vi "Check Knobs.vi"(5 "Knobs Present":bool[](array[boolean]), 7 "Number of Knobs":i32, 11 "Error In":errorcluster) -> (6 "Pass/Fail?":bool, 8 "Report Text":string, 15 "Error Out":errorcluster)   [LabVIEW 2016]
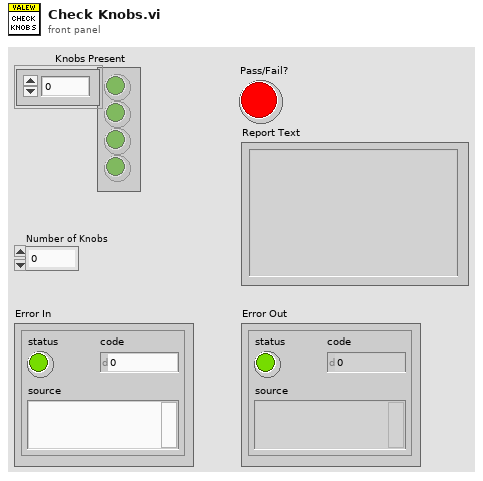
[diagram p1: front panel]
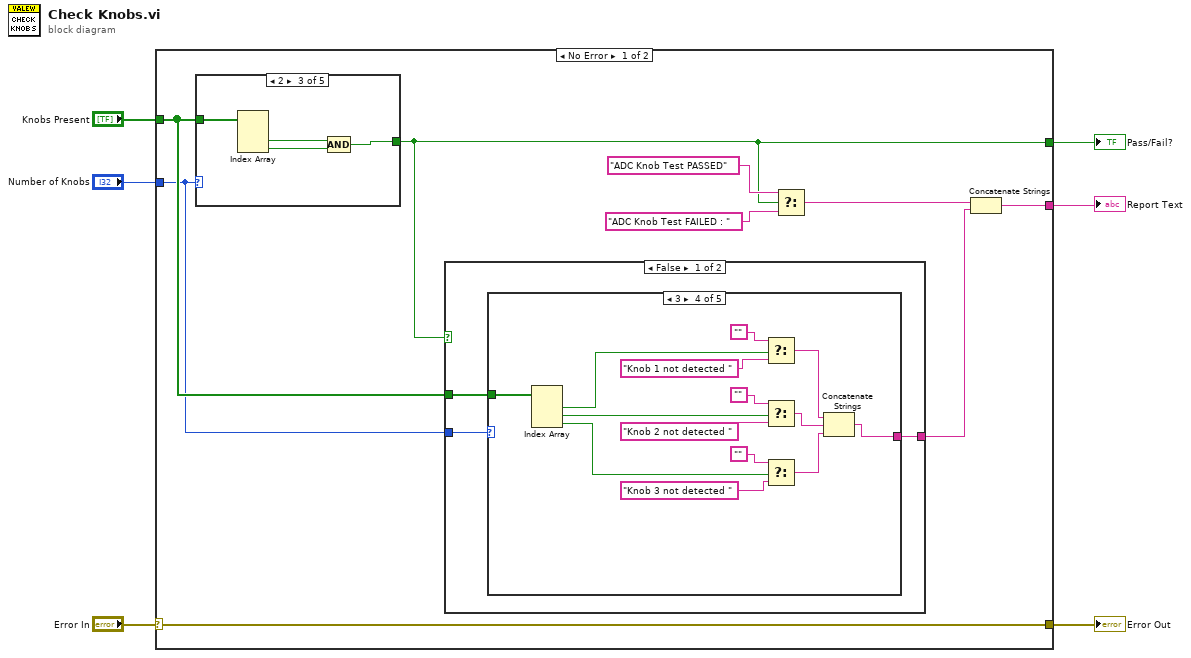
[diagram p0: block diagram]
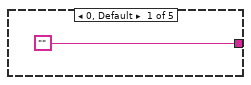
[diagram p2: hidden frame]
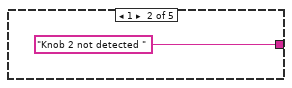
[diagram p3: hidden frame]
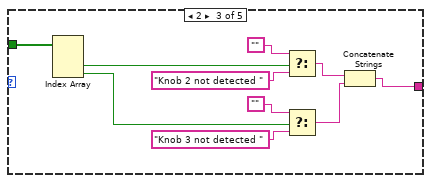
[diagram p4: hidden frame]
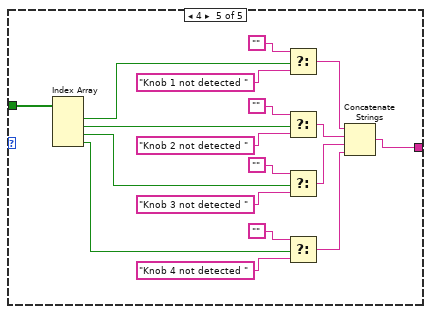
[diagram p5: hidden frame]
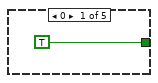
[diagram p7: hidden frame]
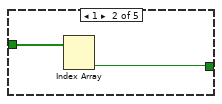
[diagram p8: hidden frame]
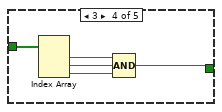
[diagram p9: hidden frame]
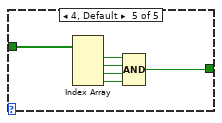
[diagram p10: hidden frame]
diagram:
  n1 = case shown="No Error" "Error In" {
    selector: "Error In" -> [w15 w81]
    tunnel: "Number of Knobs" -> [w11 _]
    tunnel: "Knobs Present" -> [w12 _]
    tunnel: [w15 w81] -> w5
    tunnel: [w9 _] -> w4
    tunnel: [w7 _] -> w3
    frame No Error {
      n2 = case shown="2" w11 {
        tunnel: w12 -> [_ w65 w69 w70 w80]
        tunnel: [TRUE ("Boolean") w64 w66 w71 w75] -> w9
        frame 0 {
        }
        frame 1 {
          n3 = Index Array(array=w65) -> (element #2=w64:bool)  [unwired: 2 in, 1 out]
        }
        frame 2 {
          n4 = Index Array(array=w69) -> (element #2=w68:bool, element #3=w67:bool)  [unwired: 3 in, 1 out]
          n5 = Compound Arithmetic op=AND(w68, w67) -> (w66:bool)
        }
        frame 3 {
          n6 = Index Array(array=w70) -> (element #1=w74:bool, element #2=w73:bool, element #3=w72:bool)  [unwired: 3 in]
          n7 = Compound Arithmetic op=AND(w74, w73, w72) -> (w71:bool)
        }
        frame 4, Default {
          n8 = Index Array(array=w80) -> (element #1=w79:bool, element #2=w78:bool, element #3=w77:bool, element #4=w76:bool)  [unwired: 4 in]
          n9 = Compound Arithmetic op=AND(w79, w78, w77, w76) -> (w75:bool)
        }
      }
      n10 = case shown="False" w9 {
        tunnel: w12 -> [w18 _]
        tunnel: w11 -> [w17 _]
        tunnel: [w16 _] -> w8
        frame False {
          n11 = case shown="3" w17 {
            tunnel: ["" "Knob 2 not detected " w22 w35 w54] -> w16
            tunnel: w18 -> [_ _ w30 w44 w62]
            frame 0, Default {
            }
            frame 1 {
            }
            frame 2 {
              n12 = Index Array(array=w30) -> (element #2=w29:bool, element #3=w24:bool)  [unwired: 3 in, 1 out]
              n13 = Select(t="", s=w29, f="Knob 2 not detected ") -> (s? t:f=w21:string)
              n14 = Select(t="", s=w24, f="Knob 3 not detected ") -> (s? t:f=w23:string)
              n15 = Concatenate Strings(w21, w23) -> (w22:string)
            }
            frame 3 {
              n16 = Index Array(array=w44) -> (element #1=w32:bool, element #2=w43:bool, element #3=w38:bool)  [unwired: 3 in]
              n17 = Select(t="", s=w32, f="Knob 1 not detected ") -> (s? t:f=w31:string)
              n18 = Select(t="", s=w43, f="Knob 2 not detected ") -> (s? t:f=w37:string)
              n19 = Select(t="", s=w38, f="Knob 3 not detected ") -> (s? t:f=w36:string)
              n20 = Concatenate Strings(w31, w37, w36) -> (w35:string)
            }
            frame 4 {
              n21 = Index Array(array=w62) -> (element #1=w51:bool, element #2=w61:bool, element #3=w57:bool, element #4=w48:bool)  [unwired: 4 in]
              n22 = Select(t="", s=w51, f="Knob 1 not detected ") -> (s? t:f=w50:string)
              n23 = Select(t="", s=w61, f="Knob 2 not detected ") -> (s? t:f=w56:string)
              n24 = Select(t="", s=w57, f="Knob 3 not detected ") -> (s? t:f=w55:string)
              n25 = Select(t="", s=w48, f="Knob 4 not detected ") -> (s? t:f=w45:string)
              n26 = Concatenate Strings(w50, w56, w55, w45) -> (w54:string)
            }
          }
        }
        frame True {
        }
      }
      n27 = Select(t="ADC Knob Test PASSED", s=w9, f="ADC Knob Test FAILED : ") -> (s? t:f=w10:string)
      n28 = Concatenate Strings(w10, w8) -> (w7:string)
    }
    frame Error {
    }
  }
  "Pass/Fail?" <- w4
  "Report Text" <- w3
  "Error Out" <- w5
